vi "Test Read.vi"() -> ()   [LabVIEW 2020]
uses:
  src/ClientApp1/ClientApp1/ClientApp1.lvclass
  C:/Users/dzoni/Documents/NJ/Playground/LV/TCP Client/client/src/ClientBase/ClientBase.lvclass
  src/ClientBase/ClientBase.lvclass
panel:
  out "ID":string
  out "Port":u16
  out "Data 2":string
  out "Data":string
  out "Address":string
  out "error out":errorcluster
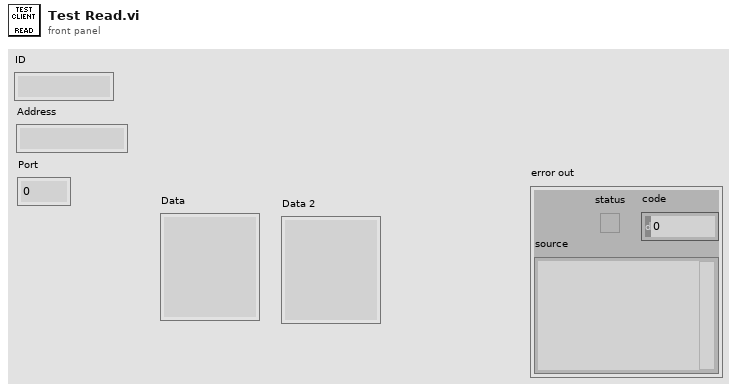
[diagram p1: front panel]
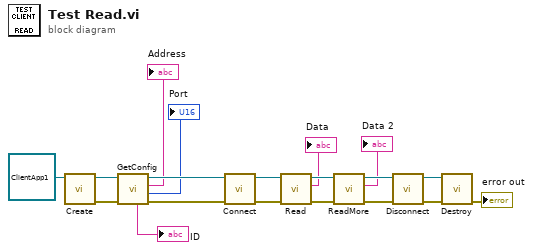
[diagram p0: block diagram]
diagram:
  n1 = call-dynamic "Create.vi"("ClientApp1 in"=refnum<class "ClientApp1.lvclass"> refnum) -> ("error out"=w10:errorcluster, "ClientApp1 out"=w13:refnum<class "ClientApp1.lvclass">)  [unwired: 9 in]
  n2 = call "GetConfig.vi"("error in (no error)"=w10, "ClientBase in"=w13) -> ("error out"=w9:errorcluster, "Port"=→"Port":u16, "Address"=→"Address":string, "ClientBase out"=w12:refnum<class "ClientApp1.lvclass">, "ID"=→"ID":string)  [unwired: 5 in]
  n3 = call-dynamic "Connect.vi"("error in (no error)"=w9, "ClientBase in"=w12) -> ("error out"=w8:errorcluster, "ClientBase out"=w11:refnum<class "ClientApp1.lvclass">)  [unwired: 8 in]
  n4 = call-dynamic "Read.vi"("error in (no error)"=w8, "ClientBase in"=w11) -> ("error out"=w7:errorcluster, "Data"=→"Data":string, "ClientBase out"=w14:refnum<class "ClientApp1.lvclass">)  [unwired: 7 in]
  n5 = call "ReadMore.vi"("error in (no error)"=w7, "ClientApp1 in"=w14) -> ("error out"=w18:errorcluster, "Data"=→"Data 2":string, "ClientApp1 out"=w19:refnum<class "ClientApp1.lvclass">)  [unwired: 7 in]
  n6 = call-dynamic "Disconnect.vi"("error in (no error)"=w18, "ClientBase in"=w19) -> ("error out"=w17:errorcluster, "ClientBase out"=w16:refnum<class "ClientApp1.lvclass">)  [unwired: 8 in]
  n7 = call-dynamic "Destroy.vi"("error in (no error)"=w17, "ClientBase in"=w16) -> ("error out"=→"error out":errorcluster)  [unwired: 9 in]
